vi "Keithley24XX_Lakeshore336_4Probe_Resistance_Controller.vi"() -> ()   [LabVIEW 2018]
uses:
  <instrlib>/Keithley 24XX/Keithley 24XX.lvlib
panel:
  out "Resistance / Differential":bool
  out "Gate Voltage":bool
  out "Program Source\nVoltage (V)":sgl
  out "Measured Src\nVoltage (V)":sgl
  out "Measured Voltage\nDifference (V)":sgl
  out "Program Gate\nVoltage (V)":sgl
  out "Measured Gate\nVoltage (V)":sgl
  out "Gate leakage \ncurrent (A)":sgl
  in  "Enabled / Disabled":bool
  out "Dup path":path
  in  "<File Name>.txt (Don't add extension)":string
  in  "Data Save Path:":path=path "C:/Users/labpc/Documents/ProbeStation Users Data"
  in  "Temperature":bool
  in  "Phase":bool
  in  "Gate Leakage Current":bool
  in  "Measurement Output":T1(radio)
  in  "Series Resistance \n(Apparatus Constant)":dbl=10000000.0
  in  "Gate\nMeasure":bool
  in  "Source \nMeasure":bool
  in  "Measurement \nDelay Time (s)":dbl=30.0
  in  "Source Voltage\nStep Time (ms) 4Probe":dbl=20.0
  in  "Source Voltage\nStep Size (V) 4Probe":dbl=0.01
  in  "Source Measurement Voltage (V)":dbl=1.0
  in  "Source Voltage \nWarmup Delay \n(Before Gate \nMeasurement)":bool
  in  "Source Voltage\nRamp On/Off":bool
  in  "Gate \nStep Time (ms)":dbl=200.0
  in  "Source Current\nCompliance Level (A)":dbl=1e-05
  in  "Source Voltage\nStep Time (ms)":dbl=200.0
  in  "Source Voltage\nStep Size (V)":dbl=0.05
  in  "Source\nVoltage Final (V)":dbl
  in  "Gate\nStep Time (ms)":dbl=200.0
  in  "Gate Voltage\nStep Size (V)":dbl=0.05
  in  "Gate \nVoltage Final (V)":dbl
  in  "Low Gate \nVoltage (V)":dbl=-80.0
  in  "Gate Voltage\nInitial Traversal Direction":enum16{"Upward", "Downward"}(ring)
  in  "Gate Voltage \nStep Size (V)":dbl=0.1
  in  "High Gate \nVoltage (V)":dbl=80.0
  in  "Gate Voltage\nInitial (V)":dbl
  in  "Gate Reset":bool
  in  "Keithley24XX Gate\nVISA resource name":refnum<visa-resource-name>="GPIB0::21::INSTR" caption="Keithley 24XX Gate\nVISA resource name"
  in  "Gate Current\nCompliance Level (A)":dbl=1.0000000005838672e-07
  in  "Source Voltage\nInitial (V)":dbl
  in  "Run Program":bool
  in  "Stop VI":bool
  in  "Source Reset":bool
  in  "Keithley24XX Source\nVISA resource name":refnum<visa-resource-name>="GPIB0::21::INSTR" caption="Keithley 24XX Source\nVISA resource name"
  in  "Program Selection":T2(radio)
  # "Welcome to Matt Gebert's Keithley / Lakeshore 4 Probe Measurement Controller.\nThis program assumes the use of two keithelys to make a 4 probe gated measurement. The Lakeshore 336 controller is optional and can be switched off.\nYou can use the different programs to:\n   1) Check current states of keithleys, \n   2) Ramp voltages to initial points for measurements, and \n   3) Perform a 4 Probe DC Gate measurement.\nThe 4 Probe measurement will sweep the range twice (ie, Up, Down) to observe hysteresis loops."
  # "LakeShore 336 Temperature Controller"
  # "Note, you  may need to set reset to TRUE to get readout working! Don't use TRUE when measuring a device! There can be voltage jumps when connected to a device and reset is on!"
  # "Keithley Source Voltage Control"
  # "Keithley Gate Voltage Control"
  # "4 Probe Output Configuration"
  # "Program: Ramp Source Voltage Configuration"
  # "Recorded Params"
  # "Output Data"
  # "Program: 4 Probe Measurement Configuration"
  # "Program: 4 Probe Measurement Configuration"
  # "Program: Ramp Gate Voltage Configuration"
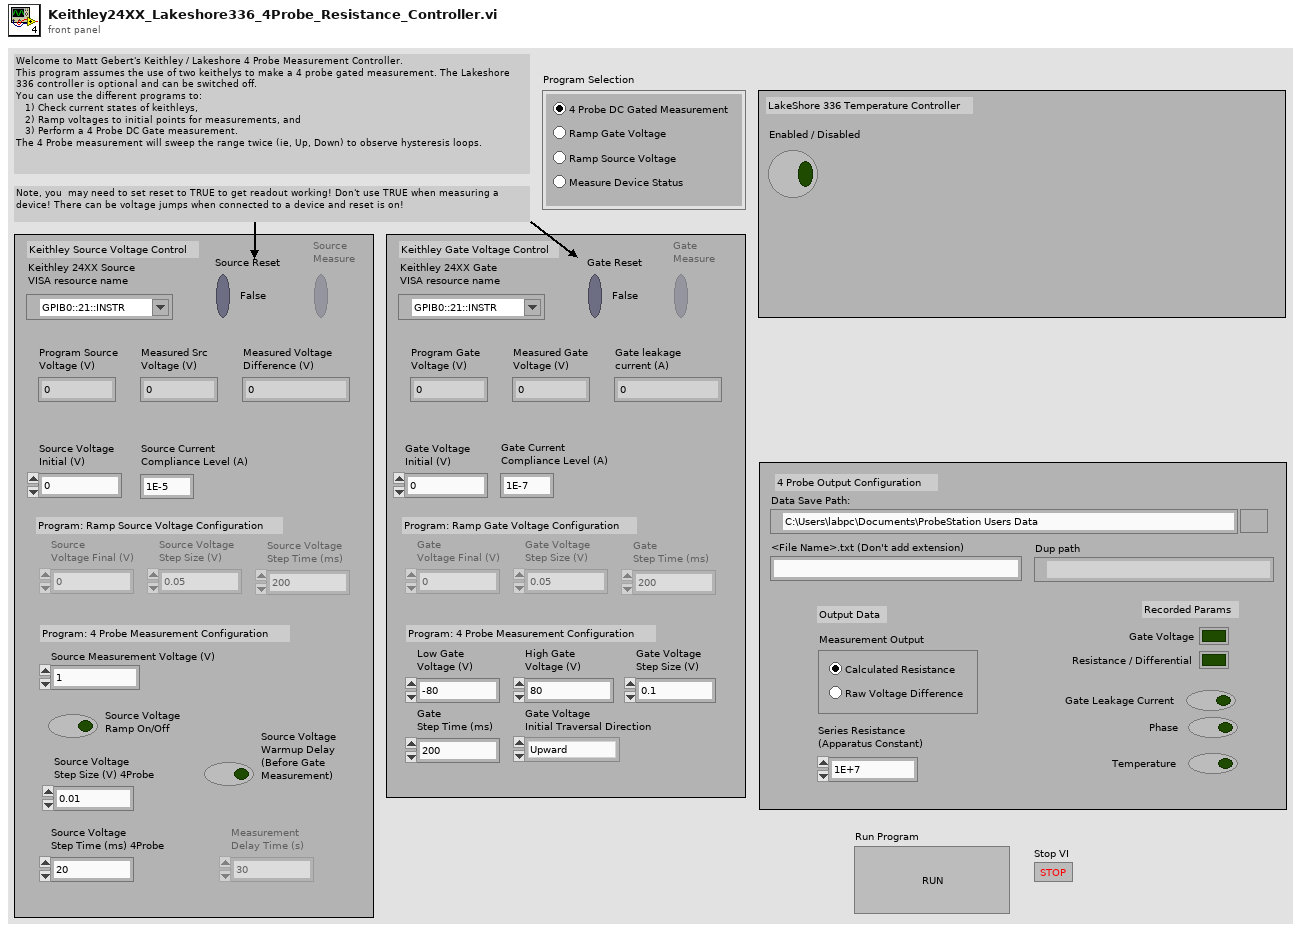
[diagram p1: front panel]
types:
  T1 = enum32{"Calculated Resistance", "Raw Voltage Difference"}
  T2 = enum32{"4 Probe Gated Measurement", "Ramp Gate Voltage", "Ramp Source Voltage", "Measure Device Status"}
  T3 = cluster{"Baud Rate":u32, "Parity":u16, "Data Bits":u16, "Stop Bits":u16, "Flow Control":u16}
  T4 = enum16{"open", "replace", "create", "open or create", "replace or create", "replace or create with confirmation"}
  T5 = enum8{"Enabled", "Disabled", "Disabled and Grayed Out"}
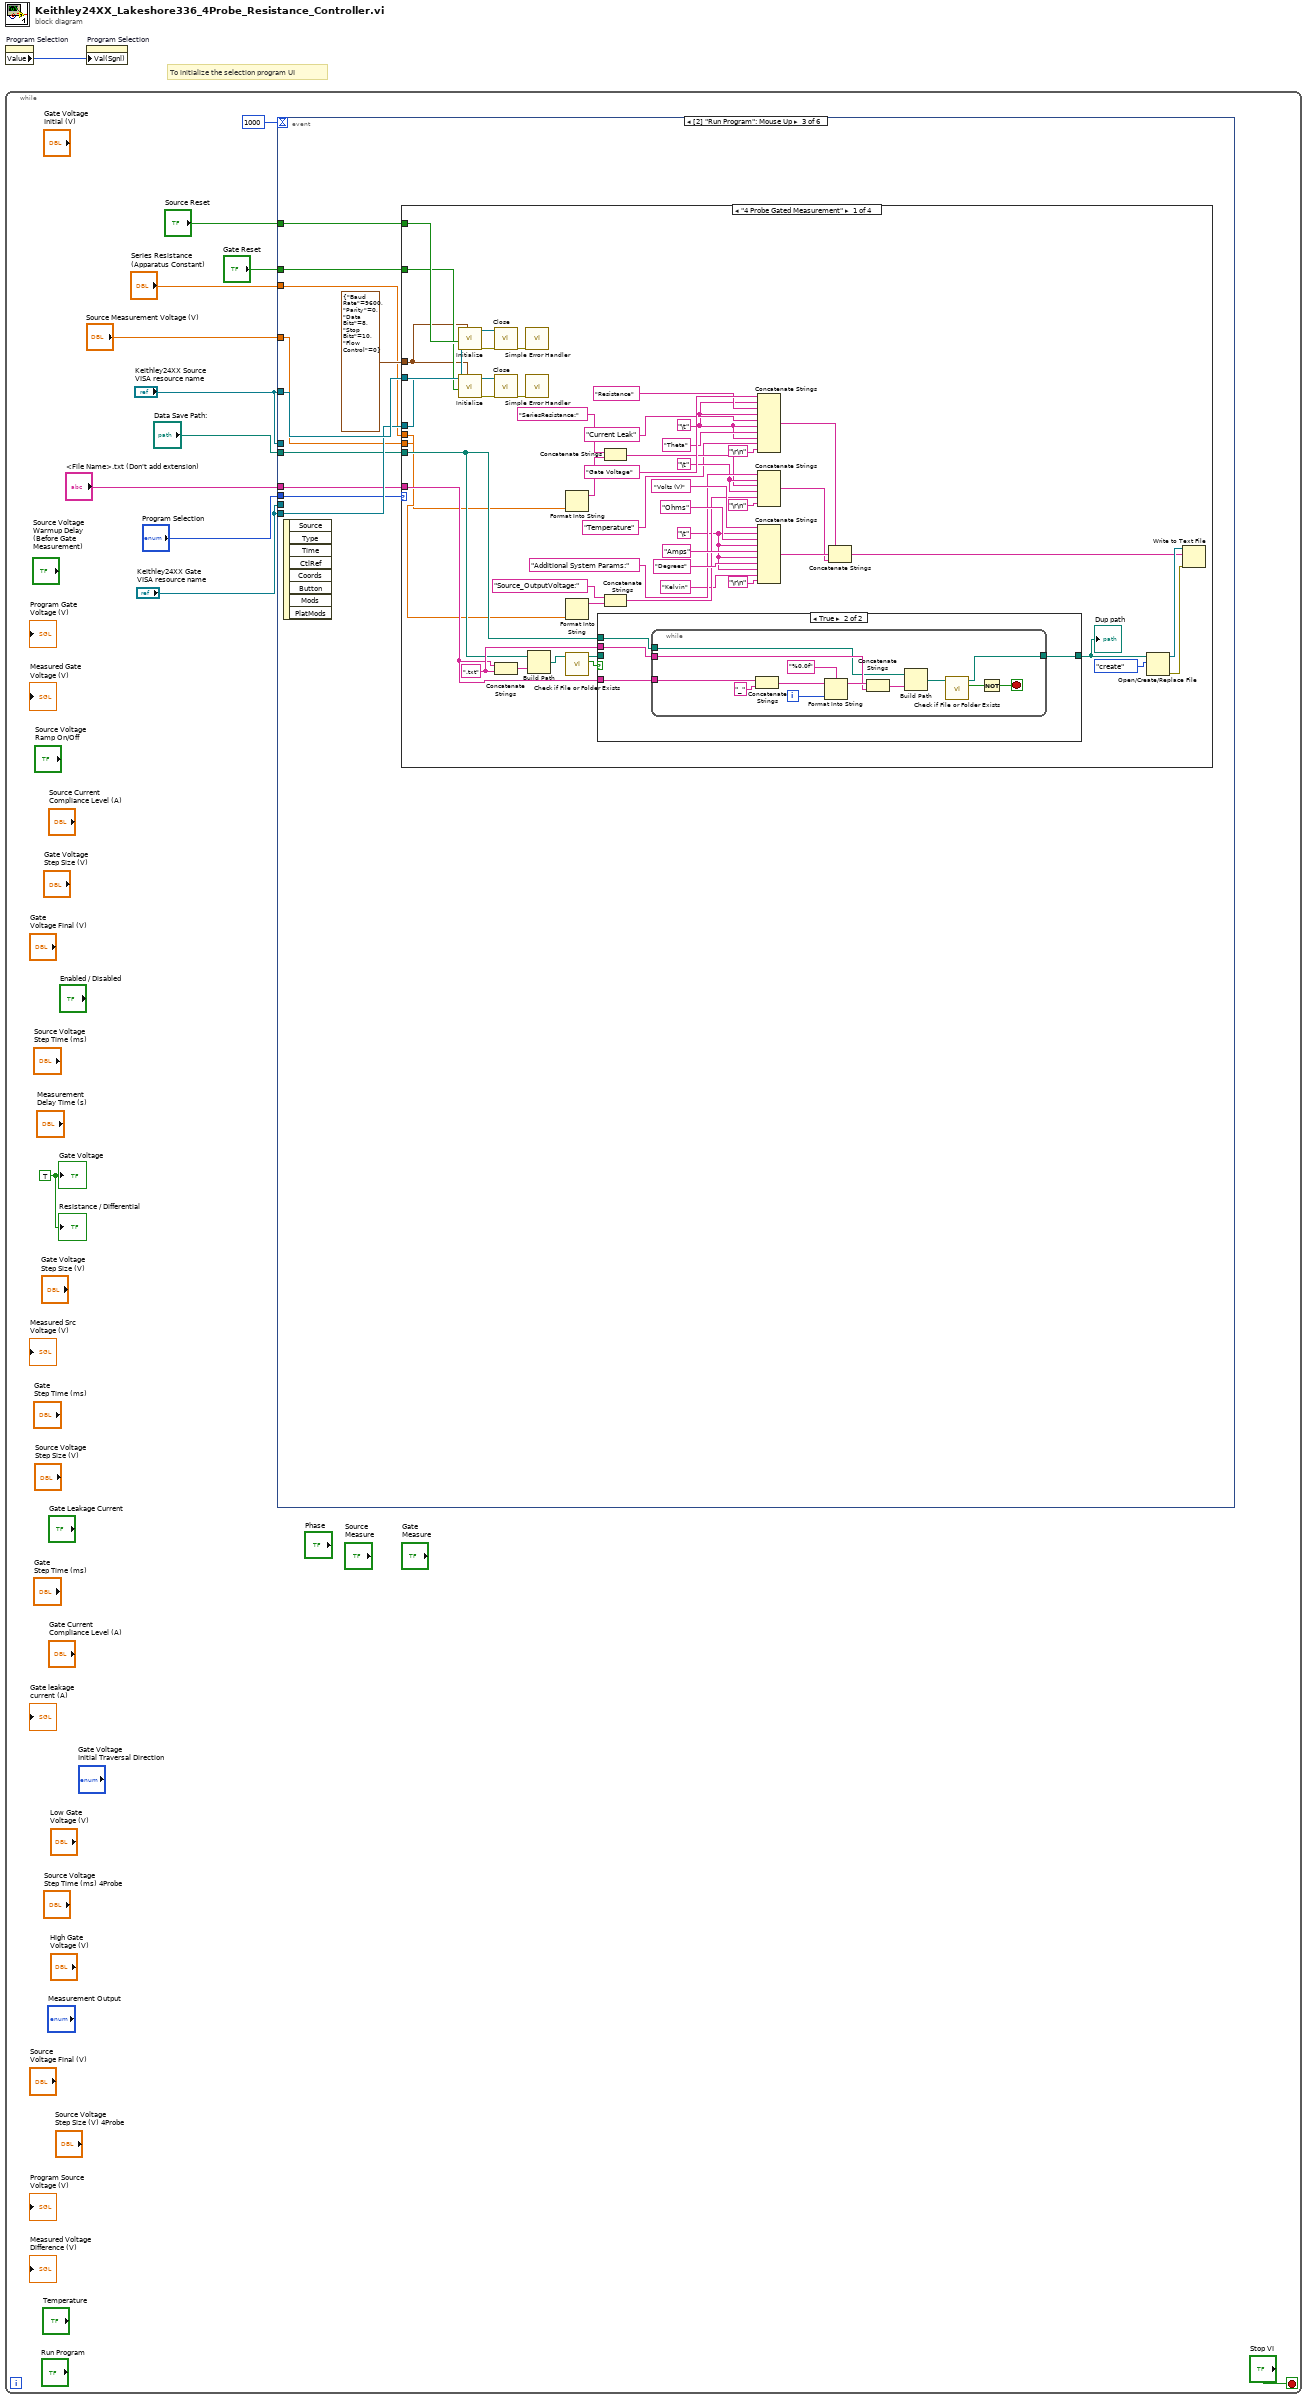
[diagram p0: block diagram]
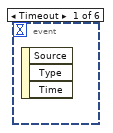
[diagram p2: hidden frame]
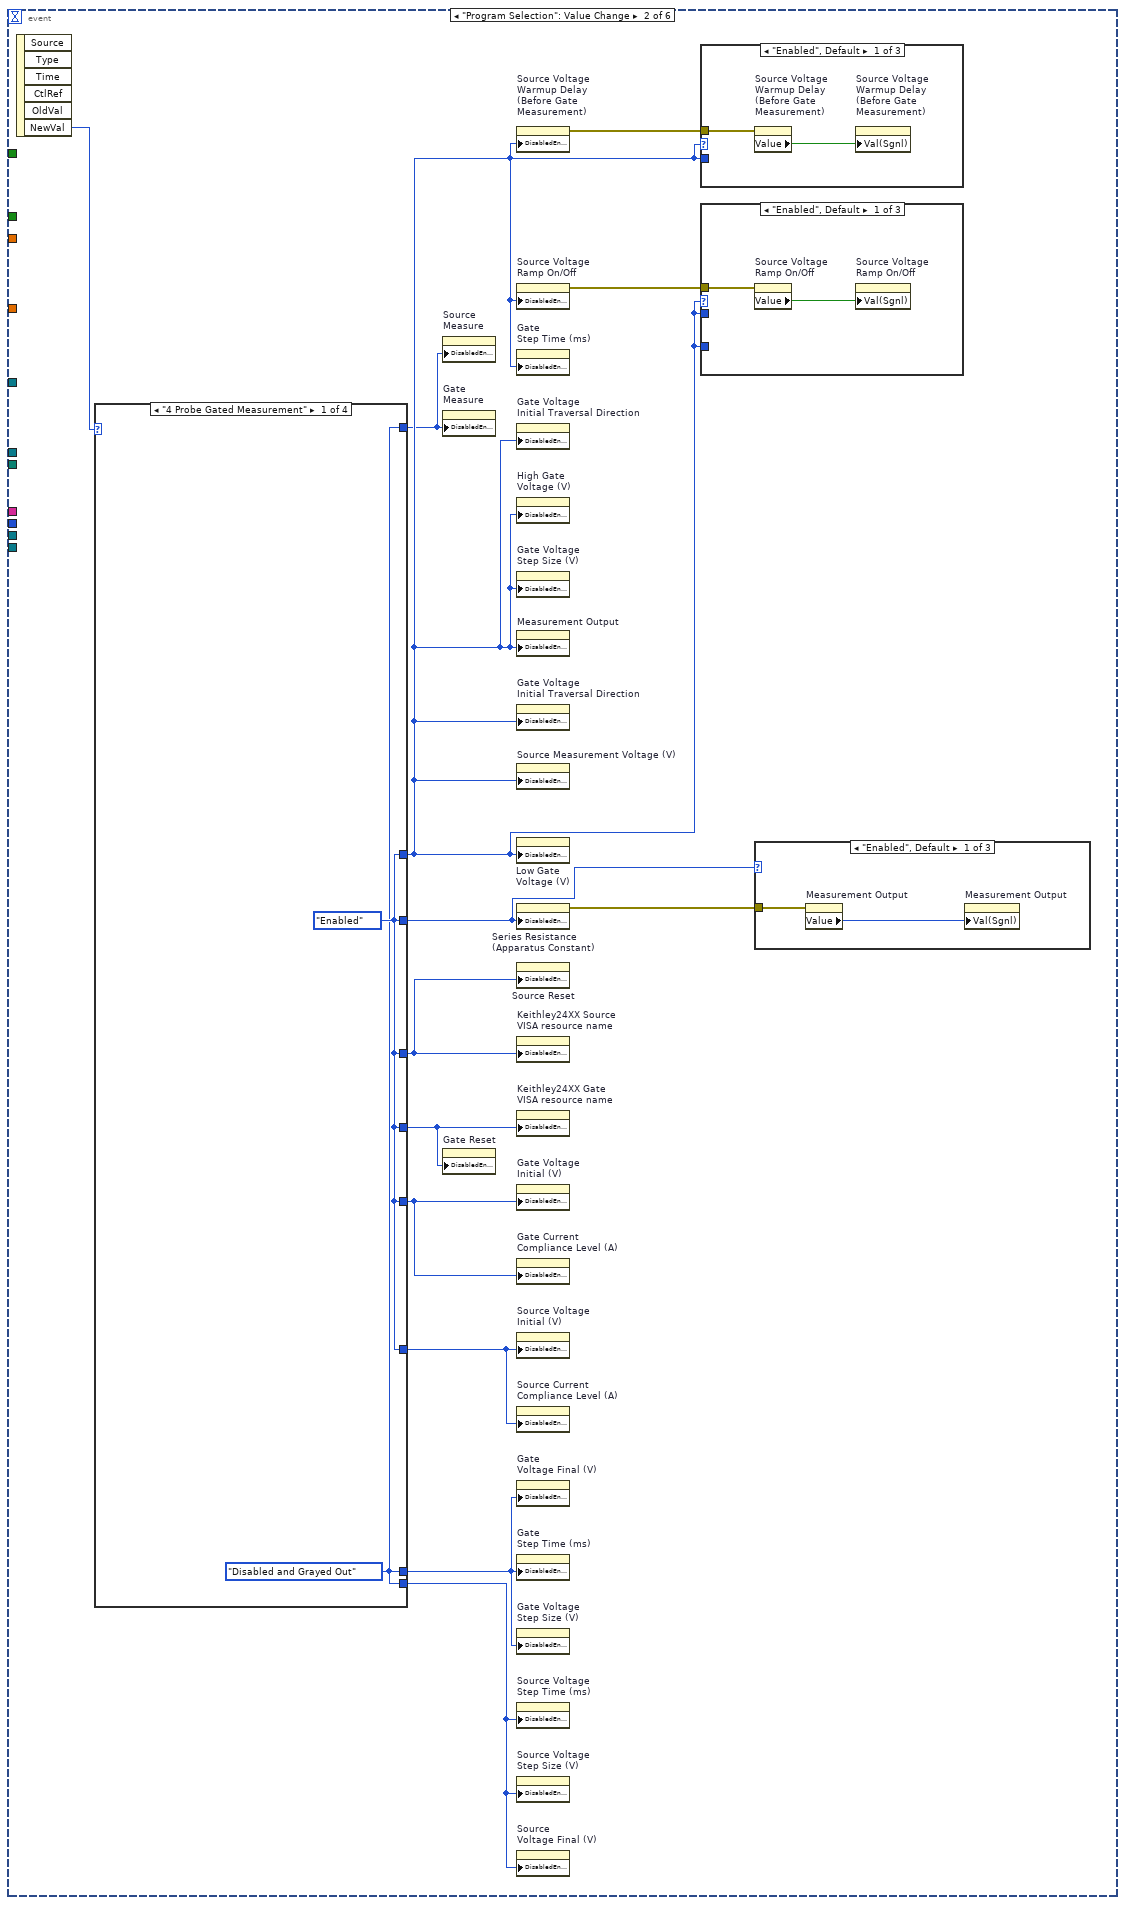
[diagram p3: hidden frame]
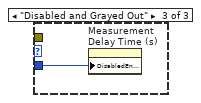
[diagram p5: hidden frame]
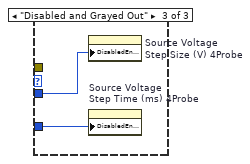
[diagram p7: hidden frame]
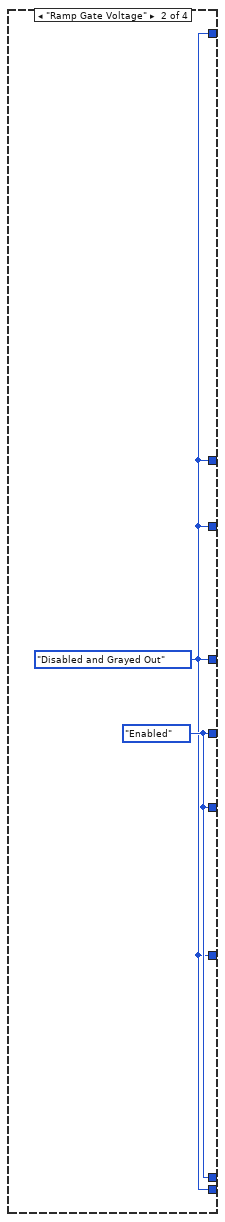
[diagram p10: hidden frame]
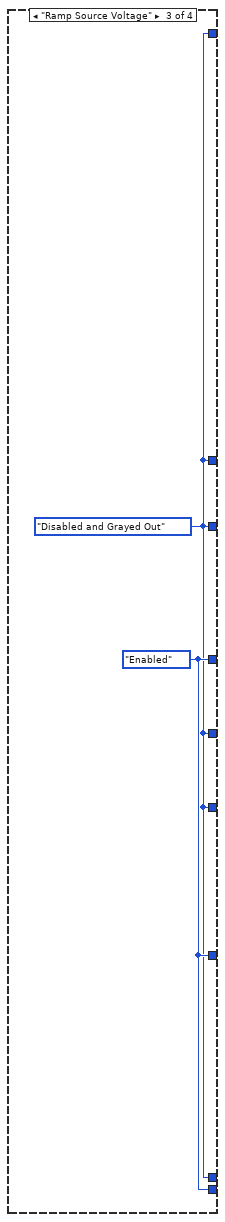
[diagram p11: hidden frame]
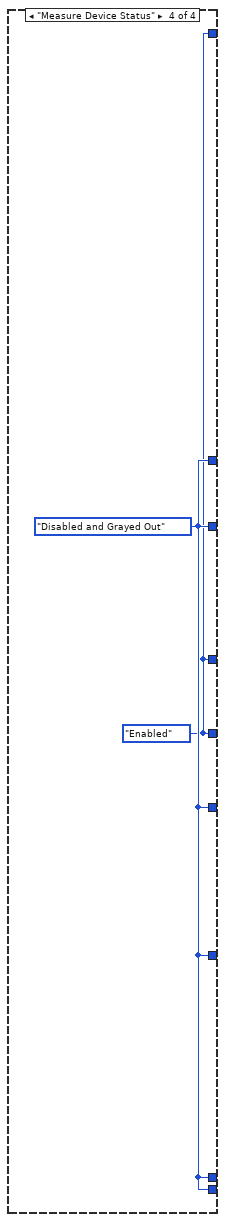
[diagram p12: hidden frame]
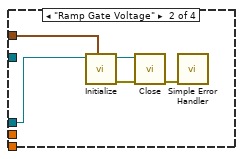
[diagram p14: hidden frame]
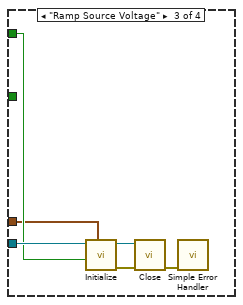
[diagram p15: hidden frame]
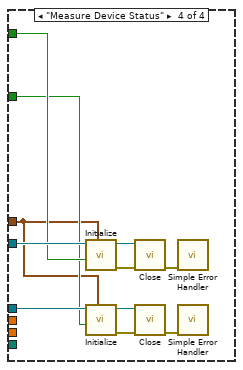
[diagram p16: hidden frame]
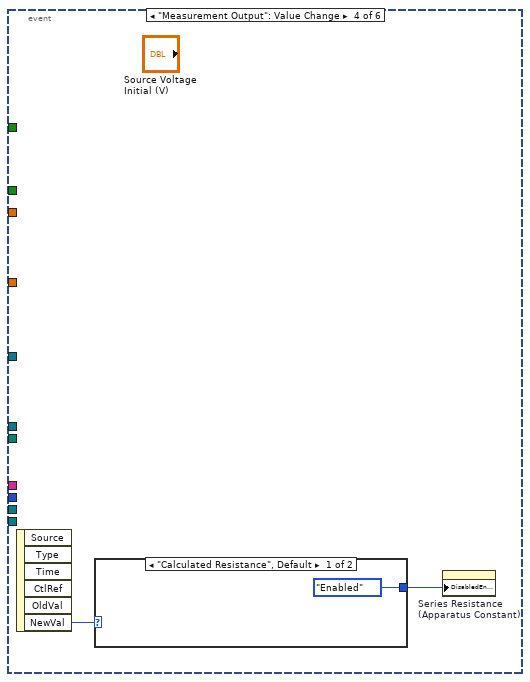
[diagram p17: hidden frame]
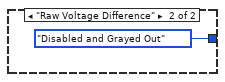
[diagram p18: hidden frame]
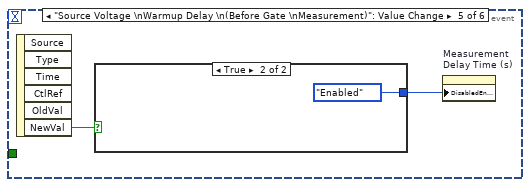
[diagram p19: hidden frame]
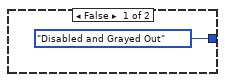
[diagram p20: hidden frame]
diagram:
  # "To initialize the selection program UI"
  n1 = property on="Program Selection" class="RadioBtnsControl (strict)"() -> ("Value"=w1:T2)  [unwired: 2 in, 2 out]
  n2 = while {
    stop <- "Stop VI" stop-if-true
    w6 = TRUE ("Gate Voltage")
    n3 = event shown="[2] \"Run Program\": Mouse Up" {
      selector: _ -> [_ _ _ _ _ _]
      dyn-events: _ -> [_ _ _ _ _ _]
      timeout: 1000 -> [_ _ _ _ _ _]
      tunnel: "Keithley24XX Gate\nVISA resource name" -> [_ _ _ _ _ _]
      tunnel: "Keithley24XX Source\nVISA resource name" -> [_ _ _ _ _ _]
      tunnel: "Source Reset" -> [_ _ w52 _ _ _]
      tunnel: "Keithley24XX Source\nVISA resource name" -> [_ _ w51 _ _ _]
      tunnel: "Gate Reset" -> [_ _ w50 _ _ _]
      tunnel: "Keithley24XX Gate\nVISA resource name" -> [_ _ w49 _ _ _]
      tunnel: "Program Selection" -> [_ _ w48 _ _ _]
      tunnel: "<File Name>.txt (Don't add extension)" -> [_ _ w47 _ _ _]
      tunnel: "Data Save Path:" -> [_ _ w46 _ _ _]
      tunnel: "Source Measurement Voltage (V)" -> [_ _ w45 _ _ _]
      tunnel: "Series Resistance \n(Apparatus Constant)" -> [_ _ w44 _ _ _]
      event Timeout {
        n4 = event-data() -> ()  [unwired: 1 in, 3 out]
      }
      event "Program Selection": Value Change {
        n5 = event-data() -> ("NewVal"=w26:T2)  [unwired: 1 in, 5 out]
        n6 = case shown="\"4 Probe Gated Measurement\"" w26 {
          tunnel: [w37 w39 w40 w42] -> w25
          tunnel: [w37 w38 w41 w42] -> w21
          tunnel: [w36 w39 w40 w43] -> w24
          tunnel: [w37 w38 w40 w43] -> w15
          tunnel: [w37 w39 w40 w43] -> w23
          tunnel: [w37 w38 w40 w43] -> w19
          tunnel: [w36 w38 w41 w43] -> w22
          tunnel: [w37 w38 w41 w43] -> w20
          tunnel: [w36 w38 w40 w42] -> w14
          frame "4 Probe Gated Measurement" {
            w36 = T5."Disabled and Grayed Out" ("Disabled")
            w37 = T5."Enabled" ("Disabled")
          }
          frame "Ramp Gate Voltage" {
            w38 = T5."Disabled and Grayed Out" ("Disabled")
            w39 = T5."Enabled" ("Disabled")
          }
          frame "Ramp Source Voltage" {
            w41 = T5."Enabled" ("Disabled")
            w40 = T5."Disabled and Grayed Out" ("Disabled")
          }
          frame "Measure Device Status" {
            w43 = T5."Disabled and Grayed Out" ("Disabled")
            w42 = T5."Enabled" ("Disabled")
          }
        }
        n7 = property on="Source \nMeasure" class="Bool (strict)"("DisabledEnum"=w14) -> ()  [unwired: 2 in, 2 out]
        n8 = property on="Gate\nMeasure" class="Bool (strict)"("DisabledEnum"=w14) -> ()  [unwired: 2 in, 2 out]
        n9 = property on="Gate Reset" class="Bool (strict)"("DisabledEnum"=w25) -> ()  [unwired: 2 in, 2 out]
        n10 = property on="Source Voltage \nWarmup Delay \n(Before Gate \nMeasurement)" class="Bool (strict)"("DisabledEnum"=w15) -> (error out=w16:errorcluster)  [unwired: 2 in, 1 out]
        n11 = property on="Source Voltage\nRamp On/Off" class="Bool (strict)"("DisabledEnum"=w15) -> (error out=w17:errorcluster)  [unwired: 2 in, 1 out]
        n12 = property on="Gate \nStep Time (ms)" class="DigNum (strict)"("DisabledEnum"=w15) -> ()  [unwired: 2 in, 2 out]
        n13 = property on="Gate Voltage\nInitial Traversal Direction" class="Enum (strict)"("DisabledEnum"=w15) -> ()  [unwired: 2 in, 2 out]
        n14 = property on="High Gate \nVoltage (V)" class="DigNum (strict)"("DisabledEnum"=w15) -> ()  [unwired: 2 in, 2 out]
        n15 = property on="Gate Voltage \nStep Size (V)" class="DigNum (strict)"("DisabledEnum"=w15) -> ()  [unwired: 2 in, 2 out]
        n16 = property on="Measurement Output" class="RadioBtnsControl (strict)"("DisabledEnum"=w15) -> ()  [unwired: 2 in, 2 out]
        n17 = property on="Gate Voltage\nInitial Traversal Direction" class="Enum (strict)"("DisabledEnum"=w15) -> ()  [unwired: 2 in, 2 out]
        n18 = property on="Source Measurement Voltage (V)" class="DigNum (strict)"("DisabledEnum"=w15) -> ()  [unwired: 2 in, 2 out]
        n19 = property on="Low Gate \nVoltage (V)" class="DigNum (strict)"("DisabledEnum"=w15) -> ()  [unwired: 2 in, 2 out]
        n20 = property on="Series Resistance \n(Apparatus Constant)" class="DigNum (strict)"("DisabledEnum"=w19) -> (error out=w18:errorcluster)  [unwired: 2 in, 1 out]
        n21 = property on="Source Reset" class="Bool (strict)"("DisabledEnum"=w21) -> ()  [unwired: 2 in, 2 out]
        n22 = property on="Keithley24XX Source\nVISA resource name" class="VISAName"("DisabledEnum"=w21) -> ()  [unwired: 2 in, 2 out]
        n23 = property on="Keithley24XX Gate\nVISA resource name" class="VISAName"("DisabledEnum"=w25) -> ()  [unwired: 2 in, 2 out]
        n24 = property on="Gate Voltage\nInitial (V)" class="DigNum (strict)"("DisabledEnum"=w23) -> ()  [unwired: 2 in, 2 out]
        n25 = property on="Gate Current\nCompliance Level (A)" class="DigNum (strict)"("DisabledEnum"=w23) -> ()  [unwired: 2 in, 2 out]
        n26 = property on="Source Voltage\nInitial (V)" class="DigNum (strict)"("DisabledEnum"=w20) -> ()  [unwired: 2 in, 2 out]
        n27 = property on="Source Current\nCompliance Level (A)" class="DigNum (strict)"("DisabledEnum"=w20) -> ()  [unwired: 2 in, 2 out]
        n28 = property on="Gate \nVoltage Final (V)" class="DigNum (strict)"("DisabledEnum"=w24) -> ()  [unwired: 2 in, 2 out]
        n29 = property on="Gate\nStep Time (ms)" class="DigNum (strict)"("DisabledEnum"=w24) -> ()  [unwired: 2 in, 2 out]
        n30 = property on="Gate Voltage\nStep Size (V)" class="DigNum (strict)"("DisabledEnum"=w24) -> ()  [unwired: 2 in, 2 out]
        n31 = property on="Source Voltage\nStep Time (ms)" class="DigNum (strict)"("DisabledEnum"=w22) -> ()  [unwired: 2 in, 2 out]
        n32 = property on="Source Voltage\nStep Size (V)" class="DigNum (strict)"("DisabledEnum"=w22) -> ()  [unwired: 2 in, 2 out]
        n33 = property on="Source\nVoltage Final (V)" class="DigNum (strict)"("DisabledEnum"=w22) -> ()  [unwired: 2 in, 2 out]
        n34 = case shown="\"Enabled\", Default" w15 {
          tunnel: w16 -> [w27 _ _]
          tunnel: w15 -> [_ _ w29]
          frame "Enabled", Default {
            n35 = property on="Source Voltage \nWarmup Delay \n(Before Gate \nMeasurement)" class="Bool (strict)"(error in=w27) -> ("Value"=w28:bool)  [unwired: 1 in, 2 out]
            n36 = property on="Source Voltage \nWarmup Delay \n(Before Gate \nMeasurement)" class="Bool (strict)"("Val(Sgnl)"=w28) -> ()  [unwired: 2 in, 2 out]
          }
          frame "Disabled" {
          }
          frame "Disabled and Grayed Out" {
            n37 = property on="Measurement \nDelay Time (s)" class="DigNum (strict)"("DisabledEnum"=w29) -> ()  [unwired: 2 in, 2 out]
          }
        }
        n38 = case shown="\"Enabled\", Default" w15 {
          tunnel: w17 -> [w30 _ _]
          tunnel: w15 -> [_ _ w33]
          tunnel: w15 -> [_ _ w32]
          frame "Enabled", Default {
            n39 = property on="Source Voltage\nRamp On/Off" class="Bool (strict)"(error in=w30) -> ("Value"=w31:bool)  [unwired: 1 in, 2 out]
            n40 = property on="Source Voltage\nRamp On/Off" class="Bool (strict)"("Val(Sgnl)"=w31) -> ()  [unwired: 2 in, 2 out]
          }
          frame "Disabled" {
          }
          frame "Disabled and Grayed Out" {
            n41 = property on="Source Voltage\nStep Size (V) 4Probe" class="DigNum (strict)"("DisabledEnum"=w32) -> ()  [unwired: 2 in, 2 out]
            n42 = property on="Source Voltage\nStep Time (ms) 4Probe" class="DigNum (strict)"("DisabledEnum"=w33) -> ()  [unwired: 2 in, 2 out]
          }
        }
        n43 = case shown="\"Enabled\", Default" w19 {
          tunnel: w18 -> [w34 _ _]
          frame "Enabled", Default {
            n44 = property on="Measurement Output" class="RadioBtnsControl (strict)"(error in=w34) -> ("Value"=w35:T1)  [unwired: 1 in, 2 out]
            n45 = property on="Measurement Output" class="RadioBtnsControl (strict)"("Val(Sgnl)"=w35) -> ()  [unwired: 2 in, 2 out]
          }
          frame "Disabled" {
          }
          frame "Disabled and Grayed Out" {
          }
        }
      }
      event "Run Program": Mouse Up {
        n46 = event-data() -> ()  [unwired: 1 in, 8 out]
        n47 = case shown="\"4 Probe Gated Measurement\"" w48 {
          tunnel: T3 {"Baud Rate"=9600, "Parity"=0, "Data Bits"=8, "Stop Bits"=10, "Flow Control"=0} ("Serial Configuration") -> [w94 w123 w128 w134]
          tunnel: w52 -> [w100 _ w129 w137]
          tunnel: w51 -> [w102 _ w130 w138]
          tunnel: w50 -> [w99 _ _ w135]
          tunnel: w49 -> [w101 w126 _ w136]
          tunnel: w47 -> [w88 _ _ _]
          tunnel: w46 -> [w87 _ _ _]
          tunnel: w45 -> [w55 _ _ _]
          tunnel: w44 -> [w54 _ _ _]
          frame "4 Probe Gated Measurement" {
            w66 = "\t"
            w58 = "\t"
            w60 = "\t"
            w89 = ".txt"
            n48 = call <instrlib>:"Initialize.vi"("Serial Configuration"=w94, "Reset (True)"=w100, "VISA resource name"=w102) -> ("error out"=w96:errorcluster, "VISA resource name out"=w104:refnum<visa-resource-name>)  [unwired: 7 in]
            n49 = call <instrlib>:"Initialize.vi"("Serial Configuration"=w94, "Reset (True)"=w99, "VISA resource name"=w101) -> ("error out"=w98:errorcluster, "VISA resource name out"=w103:refnum<visa-resource-name>)  [unwired: 7 in]
            n50 = call <instrlib>:"Close.vi"("error in (no error)"=w96, "VISA resource name"=w104) -> ("error out"=w95:errorcluster)  [unwired: 9 in]
            n51 = call <instrlib>:"Close.vi"("error in (no error)"=w98, "VISA resource name"=w103) -> ("error out"=w97:errorcluster)  [unwired: 9 in]
            n52 = Concatenate Strings(w88, w89) -> (w93:string)
            n53 = call <vilib>:"Simple Error Handler.vi"("error in (no error)"=w95) -> ()  [unwired: 4 in, 5 out]
            n54 = call <vilib>:"Simple Error Handler.vi"("error in (no error)"=w97) -> ()  [unwired: 4 in, 5 out]
            n55 = Build Path(base path=w87, name or relative path=w93) -> (appended path=w92:path)
            n56 = Format Into String(w54) -> (resulting string=w82:string)  [unwired: 3 in, 1 out]
            n57 = Format Into String(w55) -> (resulting string=w81:string)  [unwired: 3 in, 1 out]
            n58 = call <vilib>:"Check if File or Folder Exists.vi"("path"=w92) -> ("file or folder exists?"=w91:bool, "dup path"=w90:path)  [unwired: 8 in, 1 out]
            n59 = case shown="True" w91 {
              tunnel: [w105 w106] -> w83
              tunnel: w90 -> [w105 _]
              tunnel: w87 -> [_ w107]
              tunnel: w88 -> [_ w109]
              tunnel: w89 -> [_ w108]
              frame False {
              }
              frame True {
                n60 = while {
                  tunnel: w109 -> [w112]
                  tunnel: w108 -> [w117]
                  tunnel: w107 -> [w115]
                  tunnel: [w113] -> w106
                  i -> [w119]
                  stop <- w121 stop-if-true
                  n61 = Concatenate Strings(w112, "_" ("string")) -> (w111:string)
                  n62 = Format Into String(format string="%0.0f", initial string=w111, w119) -> (resulting string=w118:string)  [unwired: 1 in, 1 out]
                  n63 = Concatenate Strings(w118, w117) -> (w116:string)
                  n64 = Build Path(base path=w115, name or relative path=w116) -> (appended path=w114:path)
                  n65 = call <vilib>:"Check if File or Folder Exists.vi"("path"=w114) -> ("file or folder exists?"=w122:bool, "dup path"=w113:path)  [unwired: 8 in, 1 out]
                  n66 = Not(x=w122) -> (.not. x?=w121:bool)
                }
              }
            }
            "Dup path" <- w83
            n67 = Concatenate Strings("SeriesResistance:" ("string"), w82) -> (w65:string)
            n68 = Concatenate Strings("Source_OutputVoltage:" ("string"), w81) -> (w64:string)
            n69 = Concatenate Strings("Gate Voltage" ("string"), w60, "Resistance" ("string"), w60, "Current Leak" ("string"), w60, "Theta" ("string"), w60, "Temperature" ("string"), "\r\n") -> (w78:string)
            n70 = Concatenate Strings("Additional System Params:" ("string"), w66, w65, w66, w64, "\r\n") -> (w67:string)
            n71 = Concatenate Strings("Volts (V)" ("string"), w58, "Ohms" ("string"), w58, "Amps" ("string"), w58, "Degrees" ("string"), w58, "Kelvin" ("string"), "\r\n") -> (w77:string)
            n72 = Concatenate Strings(w78, w77, w67) -> (w56:string)
            n73 = Open/Create/Replace File(file path (use dialog)=w83, operation (0:open)=T4."create") -> (refnum out=w85:refnum<file>, error out=w84:errorcluster)  [unwired: 4 in, 1 out]
            n74 = Write to Text File(file (use dialog)=w85, text=w56, error in=w84) -> ()  [unwired: 1 in, 3 out]
          }
          frame "Ramp Gate Voltage" {
            n75 = call <instrlib>:"Initialize.vi"("Serial Configuration"=w123, "VISA resource name"=w126) -> ("error out"=w125:errorcluster, "VISA resource name out"=w127:refnum<visa-resource-name>)  [unwired: 8 in]
            n76 = call <instrlib>:"Close.vi"("error in (no error)"=w125, "VISA resource name"=w127) -> ("error out"=w124:errorcluster)  [unwired: 9 in]
            n77 = call <vilib>:"Simple Error Handler.vi"("error in (no error)"=w124) -> ()  [unwired: 4 in, 5 out]
          }
          frame "Ramp Source Voltage" {
            n78 = call <instrlib>:"Initialize.vi"("Serial Configuration"=w128, "Reset (True)"=w129, "VISA resource name"=w130) -> ("error out"=w133:errorcluster, "VISA resource name out"=w131:refnum<visa-resource-name>)  [unwired: 7 in]
            n79 = call <instrlib>:"Close.vi"("error in (no error)"=w133, "VISA resource name"=w131) -> ("error out"=w132:errorcluster)  [unwired: 9 in]
            n80 = call <vilib>:"Simple Error Handler.vi"("error in (no error)"=w132) -> ()  [unwired: 4 in, 5 out]
          }
          frame "Measure Device Status" {
            n81 = call <instrlib>:"Initialize.vi"("Serial Configuration"=w134, "Reset (True)"=w137, "VISA resource name"=w138) -> ("error out"=w141:errorcluster, "VISA resource name out"=w139:refnum<visa-resource-name>)  [unwired: 7 in]
            n82 = call <instrlib>:"Initialize.vi"("Serial Configuration"=w134, "Reset (True)"=w135, "VISA resource name"=w136) -> ("error out"=w144:errorcluster, "VISA resource name out"=w142:refnum<visa-resource-name>)  [unwired: 7 in]
            n83 = call <instrlib>:"Close.vi"("error in (no error)"=w141, "VISA resource name"=w139) -> ("error out"=w140:errorcluster)  [unwired: 9 in]
            n84 = call <instrlib>:"Close.vi"("error in (no error)"=w144, "VISA resource name"=w142) -> ("error out"=w143:errorcluster)  [unwired: 9 in]
            n85 = call <vilib>:"Simple Error Handler.vi"("error in (no error)"=w140) -> ()  [unwired: 4 in, 5 out]
            n86 = call <vilib>:"Simple Error Handler.vi"("error in (no error)"=w143) -> ()  [unwired: 4 in, 5 out]
          }
        }
      }
      event "Measurement Output": Value Change {
        n87 = event-data() -> ("NewVal"=w146:T1)  [unwired: 1 in, 5 out]
        n88 = case shown="\"Calculated Resistance\", Default" w146 {
          tunnel: [T5."Enabled" ("Disabled") T5."Disabled and Grayed Out" ("Disabled")] -> w145
          frame "Calculated Resistance", Default {
          }
          frame "Raw Voltage Difference" {
          }
        }
        n89 = property on="Series Resistance \n(Apparatus Constant)" class="DigNum (strict)"("DisabledEnum"=w145) -> ()  [unwired: 2 in, 2 out]
      }
      event "Source Voltage \nWarmup Delay \n(Before Gate \nMeasurement)": Value Change {
        n90 = event-data() -> ("NewVal"=w149:bool)  [unwired: 1 in, 5 out]
        n91 = case shown="True" w149 {
          tunnel: [T5."Disabled and Grayed Out" ("Disabled") T5."Enabled" ("Disabled")] -> w150
          frame False {
          }
          frame True {
          }
        }
        n92 = property on="Measurement \nDelay Time (s)" class="DigNum (strict)"("DisabledEnum"=w150) -> ()  [unwired: 2 in, 2 out]
      }
      event "Source Voltage\nRamp On/Off": Value Change {
        n93 = event-data() -> ("NewVal"=w153:bool)  [unwired: 1 in, 5 out]
        n94 = case shown="True" w153 {
          tunnel: [T5."Disabled and Grayed Out" ("Disabled") T5."Enabled" ("Disabled")] -> w154
          frame False {
          }
          frame True {
          }
        }
        n95 = property on="Source Voltage\nStep Time (ms) 4Probe" class="DigNum (strict)"("DisabledEnum"=w154) -> ()  [unwired: 2 in, 2 out]
        n96 = property on="Source Voltage\nStep Size (V) 4Probe" class="DigNum (strict)"("DisabledEnum"=w154) -> ()  [unwired: 2 in, 2 out]
      }
    }
    "Gate Voltage" <- w6
    "Resistance / Differential" <- w6
  }
  n97 = property on="Program Selection" class="RadioBtnsControl (strict)"("Val(Sgnl)"=w1) -> ()  [unwired: 2 in, 2 out]
